vi "niDTS Template RF Test Set Parameters.vi"(0 "Template Tx Test Handle in":T2, 7 "Parameters":T1, 11 "error in (no error)":errorcluster) -> (4 "Template Tx Test Handle out":T2, 15 "error out":errorcluster)   [LabVIEW 2014, in "niDTS Template.lvlib"]
uses:
  niDTS Template.lvlib
  Includes/Template RF Test INC Handle.ctl
  Objects/BASE_class/Template RF Test.lvclass
  Includes/Template RF Test INC Parameters.ctl
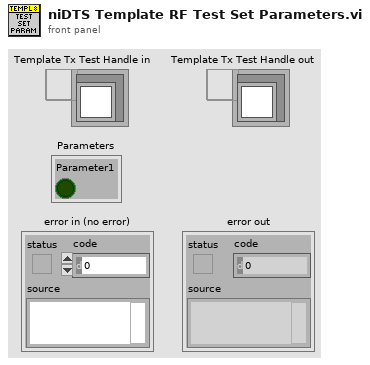
[diagram p1: front panel]
types:
  T1 = typedef "niDTS Template.lvlib/Template RF Test INC Parameters.ctl" = cluster{"Parameter1":bool}
  T2 = typedef "niDTS Template.lvlib/Template RF Test INC Handle.ctl" = refnum<data-value>
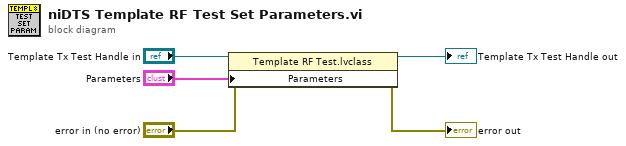
[diagram p0: block diagram]
diagram:
  n1 = property class="Template RF Test.lvclass"(reference="Template Tx Test Handle in", error in="error in (no error)", "Parameters"="Parameters") -> (reference out=→"Template Tx Test Handle out":T2, error out=→"error out":errorcluster)
